vi "Add Source Path if Error.vi"(8 "error in (no error)":errorcluster, 11 "JSON Deserializer in":refnum<class "JSON Deserializer.lvclass">) -> (0 "error out":errorcluster, 3 "JSON Deserializer out":refnum<class "JSON Deserializer.lvclass">)   [LabVIEW 2020, in "JKI JSON Serialization.lvlib" / "JSON Deserializer.lvclass"]
doc: "Add Source Path to Error description if incoming error exists."
uses:
  JSON Deserializer.lvclass
  JSON Deserializer.lvclass/JSON Deserializer.ctl
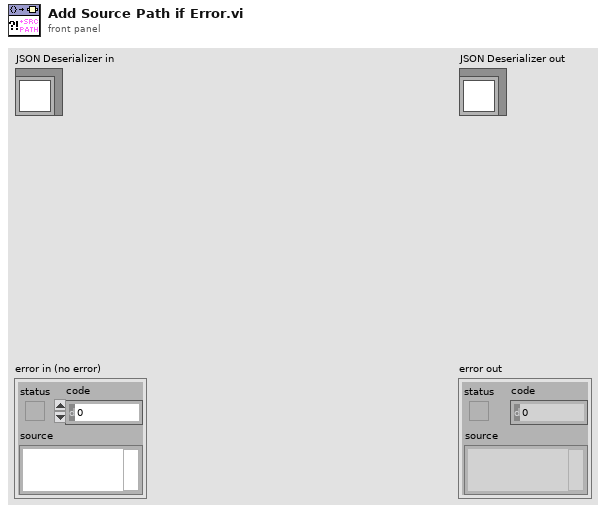
[diagram p1: front panel]
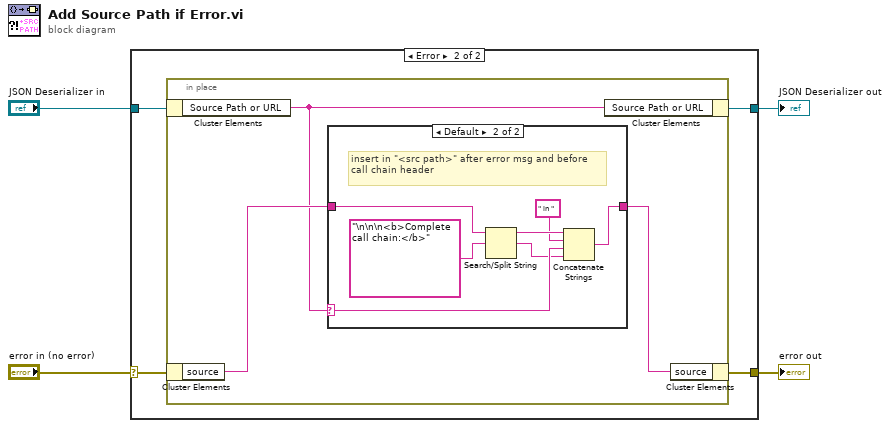
[diagram p0: block diagram]
diagram:
  n1 = case shown="Error" "error in (no error)" {
    selector: "error in (no error)" -> [w6 w10]
    tunnel: [w6 w9] -> w3
    tunnel: [w5 w7] -> w1
    tunnel: "JSON Deserializer in" -> [w5 w8]
    frame No Error {
    }
    frame Error {
      n2 = in-place {
        n3 = in-place-cluster #1(w8) -> ("Source Path or URL"=w11:string)
        n4 = in-place-cluster #2(w10) -> ("source"=w13:string)
        n5 = case shown="Default" w11 {
          selector: w11 -> [_ w17]
          tunnel: w13 -> [w14 w20]
          tunnel: [w14 w15] -> w12
          frame "" {
          }
          frame Default {
            # "insert in \"<src path>\" after error msg and before call chain header"
            n6 = Search/Split String(string=w20, search string/char (-)="\n\n\n<b>Complete call chain:</b>") -> (substring before match=w19:string, match + rest of string=w16:string)  [unwired: 1 in, 1 out]
            n7 = Concatenate Strings(w19, " in " ("string"), w17, w16) -> (w15:string)
          }
        }
        n8 = in-place-cluster #1("Source Path or URL"=w11) -> (w7:refnum<class "JSON Deserializer.lvclass">)
        n9 = in-place-cluster #2("source"=w12) -> (w9:errorcluster)
      }
    }
  }
  "error out" <- w3
  "JSON Deserializer out" <- w1
